vi "DotPoz (SubVI).vi"(10 "RangeChB":T2(ring)=enum."10 В" caption="Диапазон \"B\"", 11 "RangeChA":T1(ring)=enum."10 В" caption="Диапазон \"A\"") -> (0 "BCol":i32, 1 "ACol":i32, 2 "Chanal B":string, 3 "Chanal A":string)   [LabVIEW 2017]
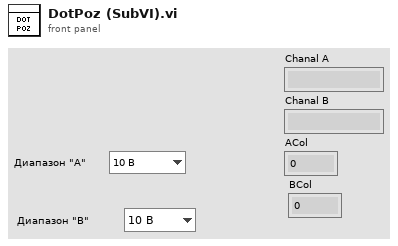
[diagram p1: front panel]
types:
  T1 = enum16{"5 мВ", "10 мВ", "25 мВ", "50 мВ", "100 мВ", "250 мВ", "0,5 В", "1,0 В", "2,5 В", "5 В", "10 В", "Авто", "Выкл."}
  T2 = enum16{"5 мВ", "10 мВ", "25 мВ", "50 мВ", "100 мВ", "250 мВ", "0,5 В", "1 В", "2,5 В", "5 В", "10 В", "Авто", "Выкл."}
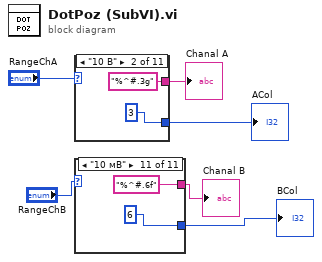
[diagram p0: block diagram]
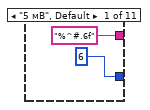
[diagram p2: hidden frame]
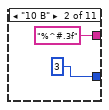
[diagram p3: hidden frame]
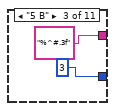
[diagram p4: hidden frame]
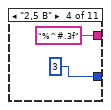
[diagram p5: hidden frame]
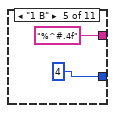
[diagram p6: hidden frame]
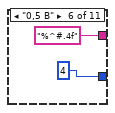
[diagram p7: hidden frame]
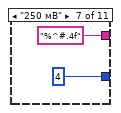
[diagram p8: hidden frame]
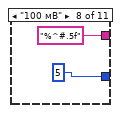
[diagram p9: hidden frame]
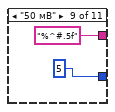
[diagram p10: hidden frame]
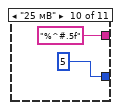
[diagram p11: hidden frame]
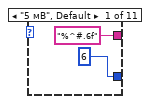
[diagram p12: hidden frame]
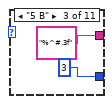
[diagram p13: hidden frame]
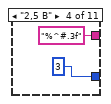
[diagram p14: hidden frame]
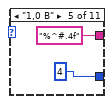
[diagram p15: hidden frame]
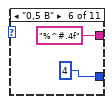
[diagram p16: hidden frame]
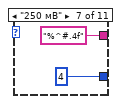
[diagram p17: hidden frame]
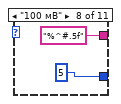
[diagram p18: hidden frame]
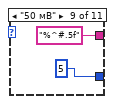
[diagram p19: hidden frame]
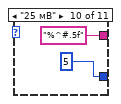
[diagram p20: hidden frame]
diagram:
  n1 = case shown="\"10 В\"" "RangeChA" {
    tunnel: ["%^#.6f" "%^#.3g" "%^#.3f" "%^#.3f" "%^#.4f" "%^#.4f" "%^#.4f" "%^#.5f" "%^#.5f" "%^#.5f" "%^#.6f"] -> w2
    tunnel: [6 3 3 3 4 4 4 5 5 5 6] -> w5
    frame "5 мВ", Default {
    }
    frame "10 В" {
    }
    frame "5 В" {
    }
    frame "2,5 В" {
    }
    frame "1,0 В" {
    }
    frame "0,5 В" {
    }
    frame "250 мВ" {
    }
    frame "100 мВ" {
    }
    frame "50 мВ" {
    }
    frame "25 мВ" {
    }
    frame "10 мВ" {
    }
  }
  "Chanal A" <- w2
  "ACol" <- w5
  n2 = case shown="\"10 мВ\"" "RangeChB" {
    tunnel: ["%^#.6f" "%^#.3f" "%^#.3f" "%^#.3f" "%^#.4f" "%^#.4f" "%^#.4f" "%^#.5f" "%^#.5f" "%^#.5f" "%^#.6f"] -> w1
    tunnel: [6 3 3 3 4 4 4 5 5 5 6] -> w3
    frame "5 мВ", Default {
    }
    frame "10 В" {
    }
    frame "5 В" {
    }
    frame "2,5 В" {
    }
    frame "1 В" {
    }
    frame "0,5 В" {
    }
    frame "250 мВ" {
    }
    frame "100 мВ" {
    }
    frame "50 мВ" {
    }
    frame "25 мВ" {
    }
    frame "10 мВ" {
    }
  }
  "Chanal B" <- w1
  "BCol" <- w3
